vi "Register for Events.vi"(8 "error in (no error)":errorcluster, 11 "Test Runner In":refnum<class "Test Runner.lvclass">) -> (0 "error out":errorcluster, 2 "Event Registration Refnum":refnum<event-registration>, 3 "Test Runner Out":refnum<class "Test Runner.lvclass">)   [LabVIEW 2020, in "Test Runner.lvclass"]
uses:
  Test Runner.lvclass
  Test Runner.lvclass/Test Runner.ctl
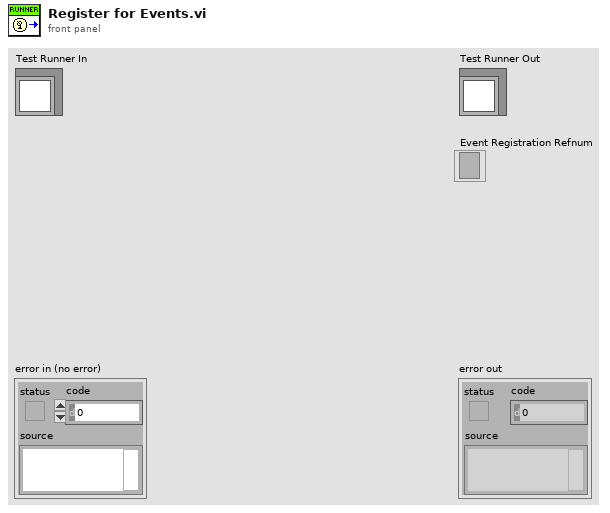
[diagram p1: front panel]
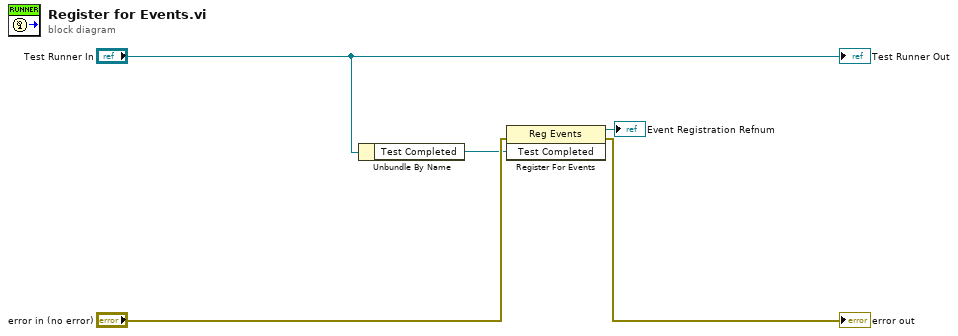
[diagram p0: block diagram]
diagram:
  n1 = Unbundle By Name("Test Runner In") -> ("Test Completed"=w2:refnum<user-event>)
  n2 = register-events(error in="error in (no error)", w2) -> (reference out=→"Event Registration Refnum":refnum<event-registration>, error out=→"error out":errorcluster)  [unwired: 1 in]
  "Test Runner Out" <- "Test Runner In"
